vi "Stage Back.vi"(8 "error in (no error)":errorcluster, 11 "Application in":refnum<class "Application.lvclass">) -> (0 "error out":errorcluster, 3 "Application out":refnum<class "Application.lvclass">)   [LabVIEW 2018, in "Application.lvlib" / "Application.lvclass"]
uses:
  Application.lvclass
  Hardware/Stage Controller/Stage Axis.ctl
  Application.lvclass/Application.ctl
  Hardware/Stage Controller Messages/Move Msg/Move Msg.lvclass/Move Msg.ctl
  <vilib>/ActorFramework/Message Enqueuer/Message Enqueuer.lvclass/Message Enqueuer.ctl
  <vilib>/ActorFramework/Message Enqueuer/Enqueue.vi
  Hardware/Stage Controller Messages/Move Msg/Move Msg.lvclass
  C:/Program Files/National Instruments/LabVIEW 2018/vi.lib/ActorFramework/Message/Message.lvclass
  <vilib>/ActorFramework/Message Priority Queue/Priority Enqueue.vi
  Hardware/Stage Controller/Stage Controller.lvclass
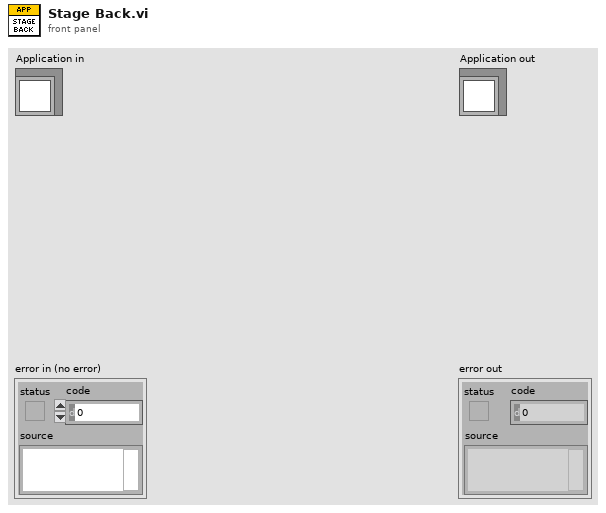
[diagram p1: front panel]
types:
  T1 = typedef "Stage Controller.lvlib/Stage Controller.lvclass/Stage Axis.ctl" = enum16{"unspecified", "X", "Y", "Z"}
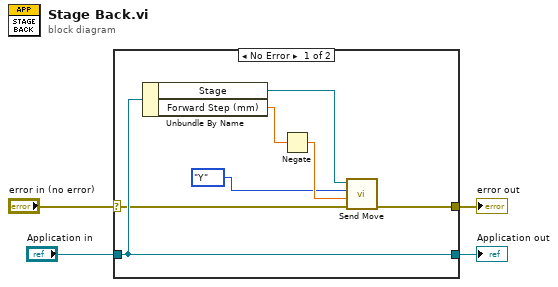
[diagram p0: block diagram]
diagram:
  n1 = case shown="No Error" "error in (no error)" {
    selector: "error in (no error)" -> [w8 w13]
    tunnel: [w9 w13] -> w3
    tunnel: [w11 w12] -> w1
    tunnel: "Application in" -> [w11 w12]
    frame No Error {
      n2 = Unbundle By Name(w11) -> ("Stage"=w10:refnum<class "Message Enqueuer.lvclass">, "Forward Step (mm)"=w7:dbl)
      n3 = Negate(x=w7) -> (-x=w6:dbl)
      n4 = call "Send Move.vi"("error in (no error)"=w8, "Distance (mm)"=w6, "Axis"=Stage_Axis."Y", "Message Enqueuer"=w10) -> ("error out"=w9:errorcluster)  [unwired: 6 in, 1 out]
    }
    frame Error {
    }
  }
  "error out" <- w3
  "Application out" <- w1
